vi "Launch Workers List.vi"() -> (0 "error out":errorcluster)   [LabVIEW 2020, in "FlexBlocks.lvlib"]
uses:
  FlexBlocks.lvlib
  Worker List UI.vi
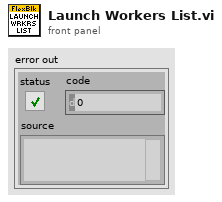
[diagram p1: front panel]
types:
  T1 = enum32{"Bad", "Idle", "Run top level", "Running"}
  T2 = enum32{"Invalid", "Standard", "Closed", "Hidden", "Minimized", "Maximized"}
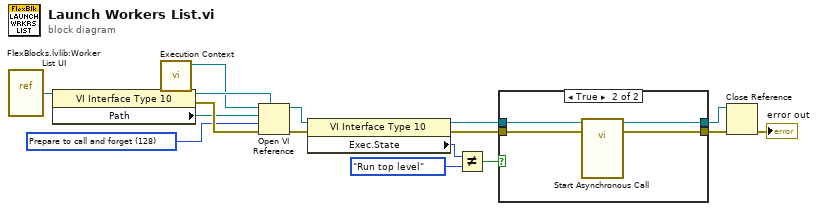
[diagram p0: block diagram]
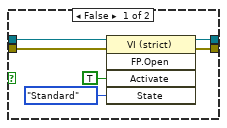
[diagram p2: hidden frame]
diagram:
  w12 = 128 items=["Record modifications"=1, "Open templates for editing"=2, "Prompt user to save"=4, "Prepare for reentrant run"=8, "Prompt to find missing subVIs"=16, "Hide loading dialog box"=32, "Enable simultaneous calls"=64, "Prepare to call and forget"=128, "Simultaneous call and forget"=192, "Prepare to call and collect"=256, "Simultaneous call and collect"=320]
  n1 = vi-ref "FlexBlocks.lvlib:Worker List UI.vi"() -> (w10:refnum<vi>)
  n2 = property class="VI Interface Type 10"(reference=w10) -> (reference out=w13:refnum<vi>, error out=w16:errorcluster, "Path"=w11:path)  [unwired: 1 in]
  n3 = call "Execution Context.vi"() -> ("Main App Instance"=w8:refnum<vi>)  [unwired: 11 in]
  n4 = Open VI Reference(type specifier VI Refnum (for type only)=w13, application reference (local)=w8, vi path=w11, options=w12, error in (no error)=w16) -> (vi reference=w6:refnum<vi>, error out=w7:errorcluster)  [unwired: 1 in]
  n5 = property class="VI Interface Type 10"(reference=w6, error in=w7) -> (reference out=w2:refnum<vi>, error out=w3:errorcluster, "Exec.State"=w5:T1)
  n6 = Not Equal?(x=w5, y=T1."Run top level") -> (x != y?=w1:bool)
  n7 = case shown="True" w1 {
    tunnel: [w20 w26] -> w15
    tunnel: [w19 w25] -> w14
    tunnel: w3 -> [w21 w24]
    tunnel: w2 -> [w22 w23]
    frame False {
      n8 = invoke class="VI (strict)" method="FP.Open"(reference=w22, error in=w21, "Activate"=TRUE ("Activate?"), "State"=T2."Standard") -> (reference out=w20:refnum<vi>, error out=w19:errorcluster)  [unwired: 1 in, 3 out]
    }
    frame True {
      n9 = call-by-ref "Start Asynchronous Call"(reference=w23, error in=w24) -> (reference out=w26:refnum<vi>, error out=w25:errorcluster)  [unwired: 12 in]
    }
  }
  n10 = Close Reference(reference=w15, error in (no error)=w14) -> (error out=→"error out":errorcluster)
